vi "Close_TextMark.vi"(0 "TextMark in":T1) -> ()   [LabVIEW 2016]
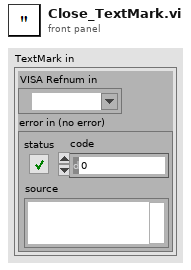
[diagram p1: front panel]
types:
  T1 = cluster{"VISA Refnum in":refnum<visa-resource-name>, "error in (no error)":errorcluster}
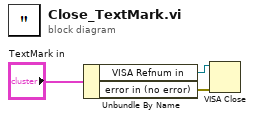
[diagram p0: block diagram]
diagram:
  n1 = Unbundle By Name("TextMark in") -> ("VISA Refnum in"=w2:refnum<visa-resource-name>, "error in (no error)"=w1:errorcluster)
  n2 = VISA Close(VISA resource name=w2, error in (no error)=w1) -> ()  [unwired: 1 out]
